vi "TiePie.CheckStatus.vi"(8 "error in (no error)":errorcluster) -> (0 "error out":errorcluster)   [LabVIEW 2014, in "LVTiePie.lvlib"]
uses:
  LVTiePie.lvlib
  bin/libtiepie.dll
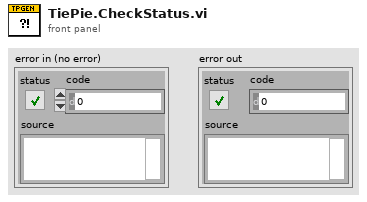
[diagram p1: front panel]
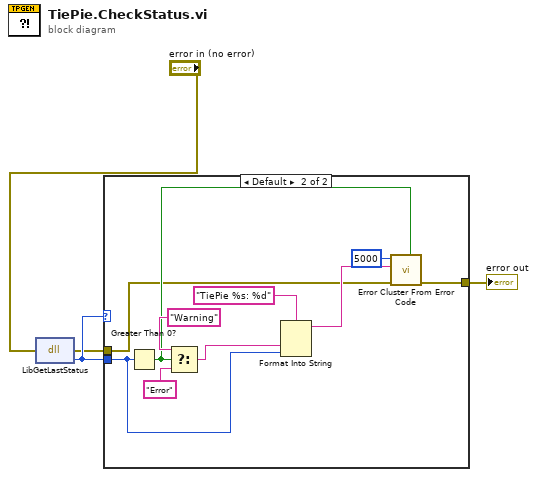
[diagram p0: block diagram]
diagram:
  n1 = dll-call lib="C:/Users/mbirski/Desktop/PAN/LabVEW/Tie Pie/bin/libtiepie.dll" fn="LibGetLastStatus"(error in="error in (no error)") -> (error out=w1:errorcluster, "return type"=w4:i32)  [unwired: 2 in, 1 out]
  n2 = case shown="Default" w4 {
    tunnel: w1 -> [w5 w8]
    tunnel: [w5 w7] -> w3
    tunnel: w4 -> [_ w6]
    frame 0 {
    }
    frame Default {
      n3 = Greater Than 0?(x=w6) -> (x > 0?=w9:bool)
      n4 = Select(t="Warning", s=w9, f="Error") -> (s? t:f=w11:string)
      n5 = Format Into String(format string="TiePie %s: %d", w11, w6) -> (resulting string=w10:string)  [unwired: 2 in, 1 out]
      n6 = call <vilib>:"Error Cluster From Error Code.vi"("is warning? (False)"=w9, "error in (no error)"=w8, "error message (\"\")"=w10, "error code (0)"=5000) -> ("error out"=w7:errorcluster)  [unwired: 5 in]
    }
  }
  "error out" <- w3
